vi "EditRow.vi"(0 "reference in":refnum<class "DataGridView.lvclass">, 5 "Row index":i32, 7 "CellValues":refnum<k24>[](array[refnum]), 11 "error in (no error)":errorcluster) -> (4 "reference out":refnum<class "DataGridView.lvclass">, 15 "error out":errorcluster)   [LabVIEW 2018, in "DataGridView.lvclass"]
doc: "Edits a row by index. the new <b>CellValues</b> will overwrite the old ones"
uses:
  DataGridView.lvclass
  System.Windows.Forms
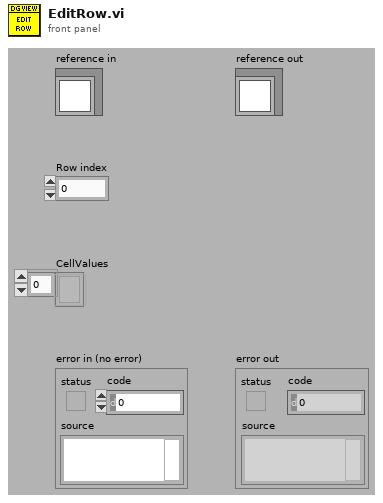
[diagram p1: front panel]
types:
  T1 = typedef "DataGridView.lvclass/ObjectAttributes.ctl" = cluster{"DataGridView":refnum<k24>, "SelectionChangedEvent":refnum<user-event>, "SelectionChanged callback ref":refnum<k27>, "LastSelectedRowIndex":i32}
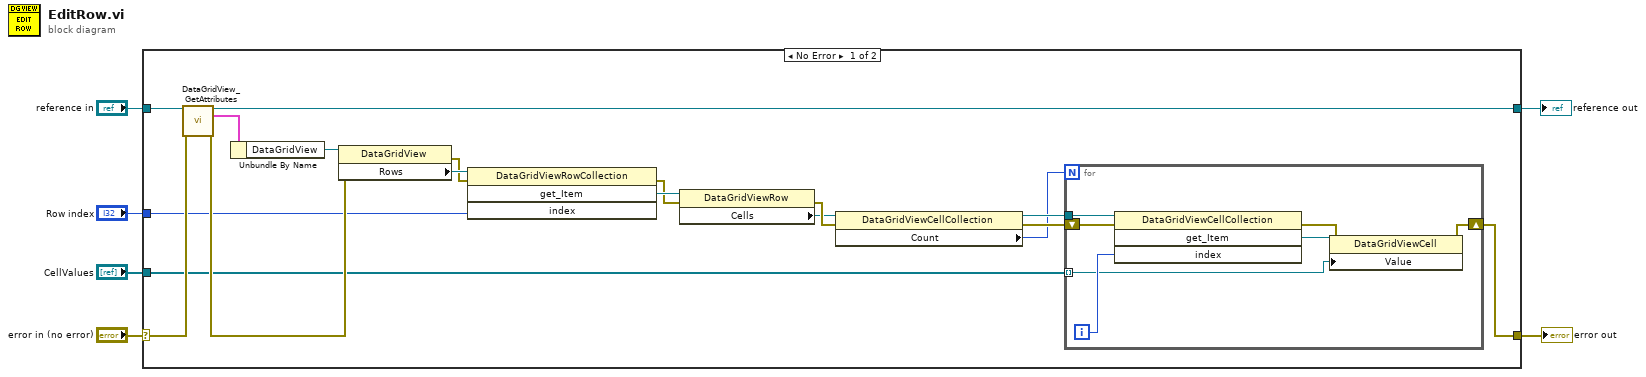
[diagram p0: block diagram]
diagram:
  n1 = case shown="No Error" "error in (no error)" {
    selector: "error in (no error)" -> [w24 w33]
    tunnel: [w21 w32] -> w4
    tunnel: "reference in" -> [w22 w32]
    tunnel: "Row index" -> [w17 _]
    tunnel: [w12 w33] -> w2
    tunnel: "CellValues" -> [w7 _]
    frame No Error {
      n2 = call "DataGridView_GetAttributes.vi"("reference in"=w22, "error in (no error)"=w24) -> ("reference out"=w21:refnum<class "DataGridView.lvclass">, "Data"=w23:T1, "error out"=w19:errorcluster)  [unwired: 10 in, 1 out]
      n3 = Unbundle By Name(w23) -> ("DataGridView"=w20:refnum<k24>)
      n4 = property class="DataGridView"(reference=w20, error in=w19) -> (error out=w15:errorcluster, "Rows"=w18:refnum<k24>)  [unwired: 1 out]
      n5 = invoke class="DataGridViewRowCollection" method="get_Item"(reference=w18, error in=w15, "index"=w17) -> (error out=w14:errorcluster, "get_Item"=w16:refnum<k24>)  [unwired: 1 in, 2 out]
      n6 = property class="DataGridViewRow"(reference=w16, error in=w14) -> (error out=w13:errorcluster, "Cells"=w10:refnum<k24>)  [unwired: 1 out]
      n7 = property class="DataGridViewCellCollection"(reference=w10, error in=w13) -> (reference out=w9:refnum<k24>, error out=w11:errorcluster, "Count"=w8:i32)
      n8 = for {
        N: w8 -> [_]
        tunnel: w9 -> [w29]
        shift-right: [w26] -> w12
        shift-left: w11 -> [w30]
        tunnel: w7 -> [w25] mode=indexing
        i -> [w28]
        n9 = invoke class="DataGridViewCellCollection" method="get_Item"(reference=w29, error in=w30, "index"=w28) -> (error out=w27:errorcluster, "get_Item"=w31:refnum<k24>)  [unwired: 1 in, 2 out]
        n10 = property class="DataGridViewCell"(reference=w31, error in=w27, "Value"=w25) -> (error out=w26:errorcluster)  [unwired: 1 out]
      }
    }
    frame Error {
    }
  }
  "error out" <- w2
  "reference out" <- w4
